vi "Assemble Subarray.vi"(8 "error in":errorcluster, 10 "message fields":T1 {"data" format="%x"; "extra" format="%x"; "msgopt" format="%04x"; "msgflag" format="%04x"; "bus" items=["BUSA", "BUSB", "BUSNONE"]; "cwd1" format="%04x"; "cwd2" format="%04x"; "swd1" format="%04x"; "swd2" format="%04x"}, 11 "message":T2) -> (0 "error out":errorcluster, 2 "subarray":dbl[](array[numeric]), 3 "value indexes":i32[](array[numeric]))   [LabVIEW 2020, in "AIM MIL-STD-1553 Engine.lvlib" / "Implementation.lvlib" / "Rx Execution Unit.lvclass"]
uses:
  Rx Execution Unit.lvclass
  Shared/Address.ctl
  Shared/Terminal Endpoint.ctl
  Shared/Parameter Definition.ctl
  Shared/Message Type.ctl
  Shared/Message Definition.ctl
  Message Map Value.ctl
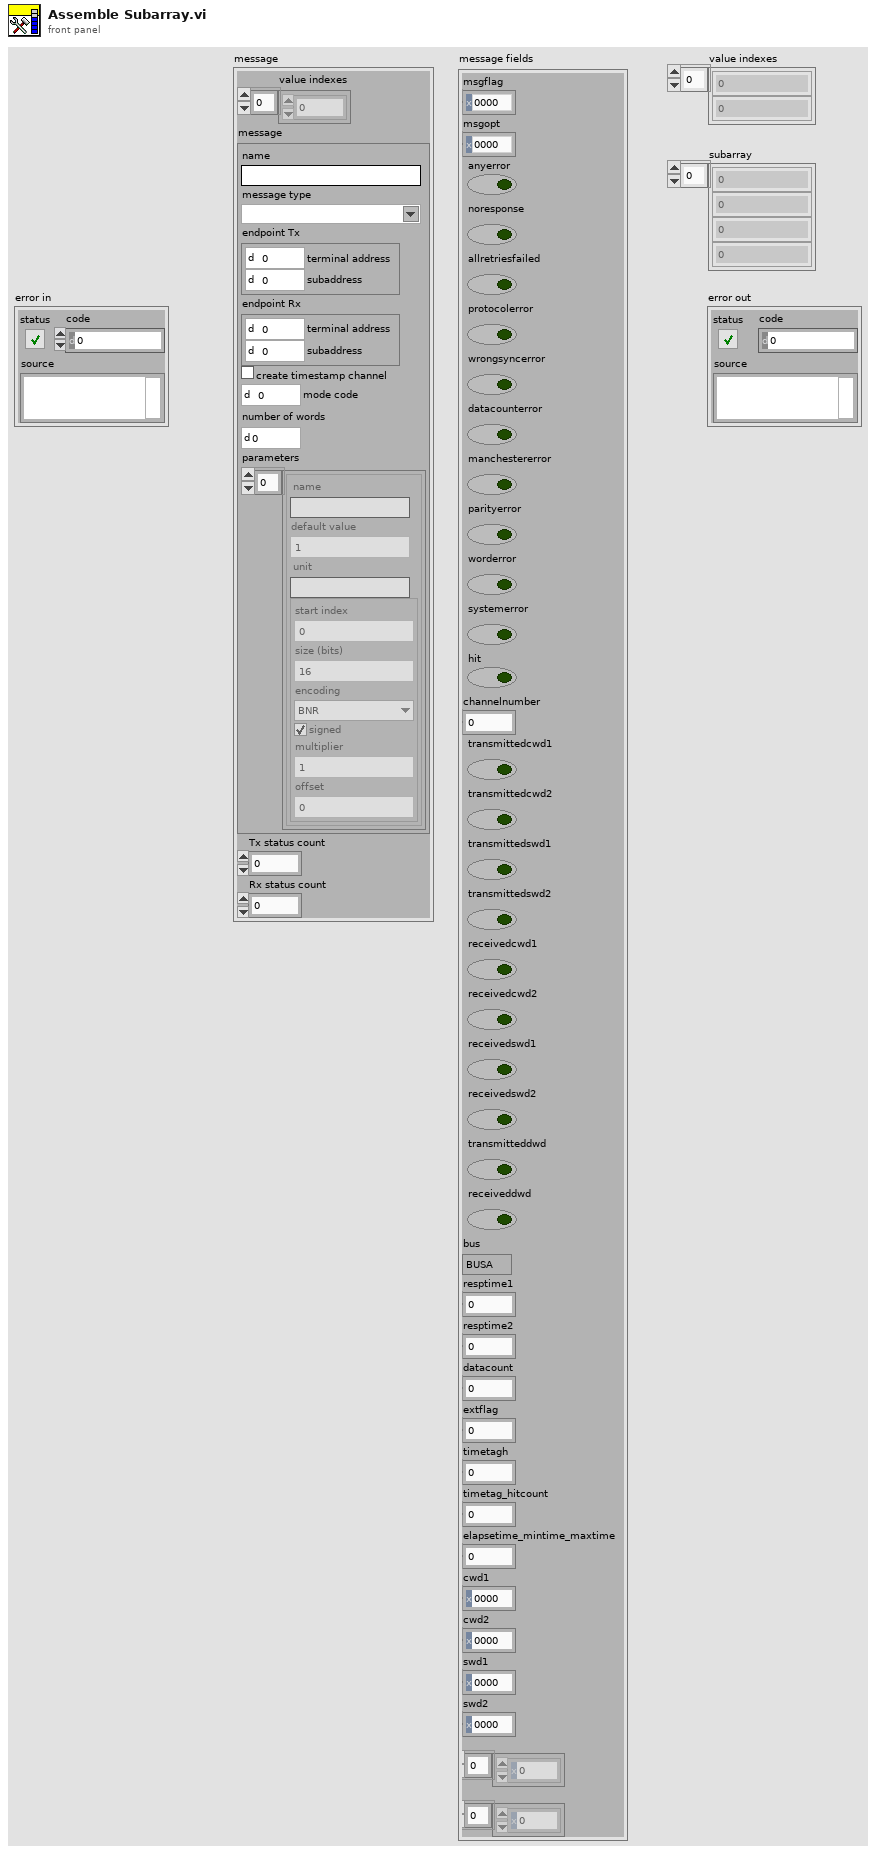
[diagram p1: front panel]
types:
  T1 = cluster{"msgflag":u16, "msgopt":u16, "anyerror":bool, "noresponse":bool, "allretriesfailed":bool, "protocolerror":bool, "wrongsyncerror":bool, "datacounterror":bool, "manchestererror":bool, "parityerror":bool, "worderror":bool, "systemerror":bool, "hit":bool, "reserved":u8, "channelnumber":i32, "transmittedcwd1":bool, "transmittedcwd2":bool, "transmittedswd1":bool, "transmittedswd2":bool, "receivedcwd1":bool, "receivedcwd2":bool, "receivedswd1":bool, "receivedswd2":bool, "transmitteddwd":bool, "receiveddwd":bool, "reserved":i8, "reserved":i8, "bus":u32, "resptime1":u16, "resptime2":u16, "datacount":u16, "extflag":u16, "timetagh":u32, "timetag_hitcount":u32, "elapsetime_mintime_maxtime":u32, "cwd1":u16, "cwd2":u16, "swd1":u16, "swd2":u16, "data":u16[], "extra":u16[]}
  T2 = typedef "AIM MIL-STD-1553 Engine.lvlib/Implementation.lvlib/Rx Execution Unit.lvclass/Message Map Value.ctl" = cluster{"value indexes":i32[], "message":T3, "Tx status count":i32, "Rx status count":i32}
  T3 = typedef "Message Definition.ctl" = cluster{"name":string, "message type":T4, "endpoint Tx":T5, "endpoint Rx":T5, "create timestamp channel":bool, "mode code":u16, "number of words":u16, "parameters":cluster{"name":string, "default value":dbl, "unit":string, "parameter definition":T7}[]}
  T4 = typedef "Message Type.ctl" = string
  T5 = typedef "Terminal Endpoint.ctl" = cluster{"terminal address":T6, "subaddress":T6}
  T6 = typedef "Address.ctl" = u16
  T7 = typedef "Parameter Definition.ctl" = cluster{"start index":i32, "size (bits)":i32, "encoding":enum16{"BNR", "BCD", "Discrete"}, "signed":bool, "multiplier":dbl, "offset":dbl}
  T8 = cluster{"name":string, "default value":dbl, "unit":string, "parameter definition":T7}[]
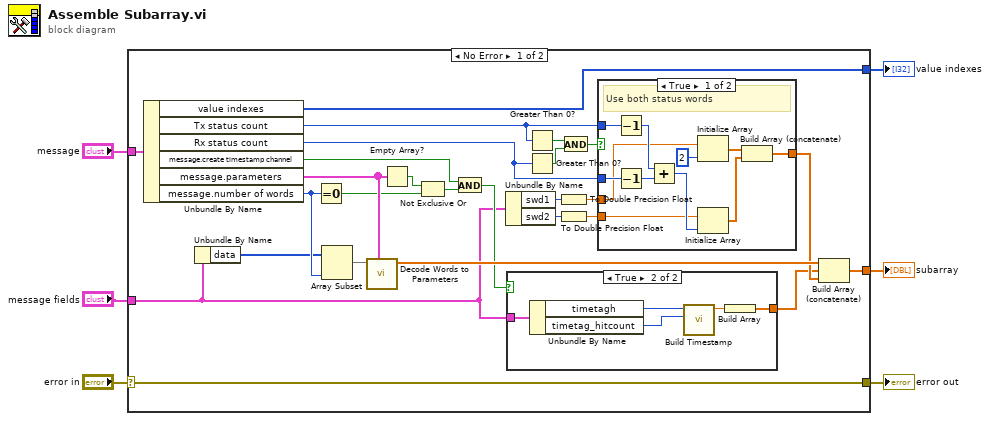
[diagram p0: block diagram]
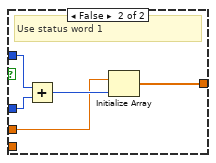
[diagram p3: hidden frame]
diagram:
  n1 = case shown="No Error" "error in" {
    selector: "error in" -> [w17 w54]
    tunnel: "message" -> [w31 _]
    tunnel: [w30 _] -> w5
    tunnel: [w19 _] -> w4
    tunnel: [w17 w54] -> w2
    tunnel: "message fields" -> [w7 _]
    frame No Error {
      n2 = Unbundle By Name(w31) -> ("value indexes"=w19:i32[], "Tx status count"=w20:i32, "Rx status count"=w21:i32, "message.create timestamp channel"=w10:bool, "message.parameters"=w15:T8, "message.number of words"=w14:u16)
      n3 = Unbundle By Name(w7) -> ("data"=w8:u16[])
      n4 = Equal To 0?(x=w14) -> (x = 0?=w12:bool)
      n5 = Array Subset(array=w8, length=w14) -> (w16:u16[])  [unwired: 1 in]
      n6 = call "Decode Words to Parameters.vi"("parameters"=w15, "data words"=w16) -> ("Values"=w32:dbl[])  [unwired: 9 in]
      n7 = Empty Array?(array=w15) -> (empty?=w13:bool)
      n8 = Not Exclusive Or(1:w12, 2:w13) -> (0:w11:bool)
      n9 = And(x=w10, y=w11) -> (x .and. y?=w9:bool)
      n10 = Unbundle By Name(w7) -> ("swd1"=w23:u16, "swd2"=w22:u16)
      n11 = case shown="True" w9 {
        tunnel: [_ w36] -> w18
        tunnel: w7 -> [_ w35]
        frame False {
        }
        frame True {
          n12 = Unbundle By Name(w35) -> ("timetagh"=w34:u32, "timetag_hitcount"=w33:u32)
          n13 = call "Build Timestamp.vi"("timestamp low bits"=w33, "timestamp high bits"=w34) -> ("timestamp out"=w37:dbl)  [unwired: 9 in]
          n14 = Build Array(w37) -> (w36:dbl[])
        }
      }
      n15 = Greater Than 0?(x=w20) -> (x > 0?=w25:bool)
      n16 = Greater Than 0?(x=w21) -> (x > 0?=w24:bool)
      n17 = To Double Precision Float(number=w23) -> (double precision float=w27:dbl)
      n18 = To Double Precision Float(number=w22) -> (double precision float=w28:dbl)
      n19 = And(x=w25, y=w24) -> (x .and. y?=w26:bool)
      n20 = case shown="True" w26 {
        tunnel: w21 -> [w45 w52]
        tunnel: [w48 w51] -> w29
        tunnel: w20 -> [w40 w50]
        tunnel: w27 -> [w39 w49]
        tunnel: w28 -> [w38 _]
        frame True {
          # "Use both status words"
          n21 = Decrement(x=w40) -> (x-1=w43:i32)
          n22 = Decrement(x=w45) -> (x-1=w44:i32)
          n23 = Add(x=w43, y=w44) -> (x+y=w41:i32)
          n24 = Initialize Array(w39, 2 ("dimension size")) -> (w47:dbl[])
          n25 = Initialize Array(w38, w41) -> (w42:dbl[])
          n26 = Build Array (concatenate)(w47, w42) -> (w48:dbl[])
        }
        frame False {
          # "Use status word 1"
          n27 = Add(x=w50, y=w52) -> (x+y=w53:i32)
          n28 = Initialize Array(w49, w53) -> (w51:dbl[])
        }
      }
      n29 = Build Array (concatenate)(w32, w18, w29) -> (w30:dbl[])
    }
    frame Error {
    }
  }
  "subarray" <- w5
  "value indexes" <- w4
  "error out" <- w2
